vi "UIDisable.vi"(1 "数组":refnum<vi>[](array[refnum])) -> ()   [LabVIEW 2018]
uses:
  Device VIs/Verbal.vi
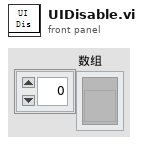
[diagram p1: front panel]
types:
  T1 = enum8{"Enabled", "Disabled", "Disabled and Grayed Out"}
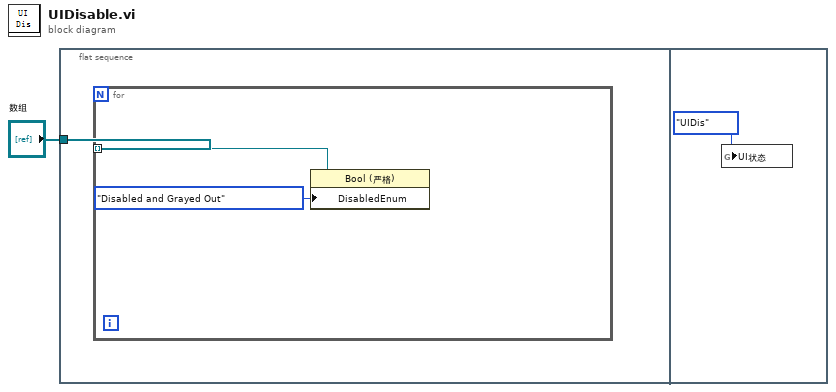
[diagram p0: block diagram]
diagram:
  n1 = flat-sequence {
    tunnel: "数组" -> [w2]
    frame #0 {
      n2 = for {
        tunnel: w2 -> [w4] mode=indexing
        n3 = property class="Bool (严格)"(reference=w4, "DisabledEnum"=T1."Disabled and Grayed Out" ("禁用")) -> ()  [unwired: 1 in, 2 out]
      }
    }
    frame #1 {
      n4 = global write "Verbal.vi" "UI状态"(enum16{"UIEn", "UIDis"}."UIDis" ("UI状态")) -> ()
    }
  }
